vi "TCP - Engine Sender Queue Driver.vi"(6 "timeout(ms)":i32=-1, 7 "Cases":T2, 8 "error in (no error)":errorcluster, 10 "Element In":cluster{"Data":variant, "State":T1}={"Data"=variant, "State"=enum."Boolean Commands"}) -> (0 "error out":errorcluster, 2 "Element Out":cluster{"Data":variant, "State":T1}={"Data"=variant, "State"=enum."Boolean Commands"}, 3 "queue out":refnum<queue>)   [LabVIEW 2017]
uses:
  TCP - Driver Control.ctl
  Controls/RT- Queue States.ctl
panel:
  in  "Enum":T1
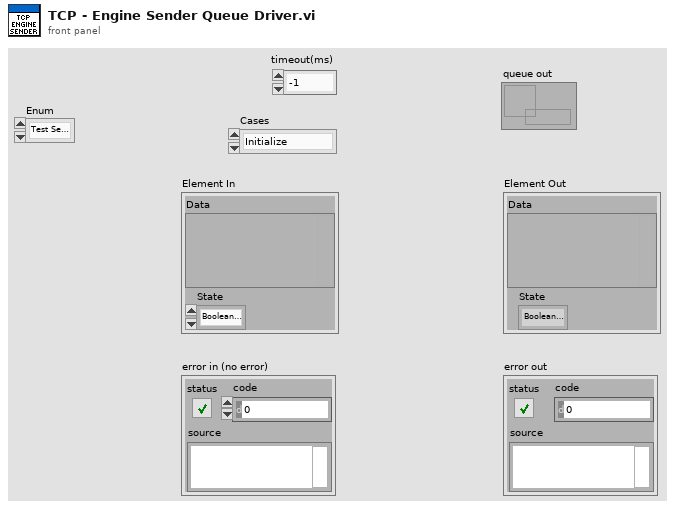
[diagram p1: front panel]
types:
  T1 = typedef "TCP - Driver Control.ctl" = enum16{"Test Settings", "Boolean Commands", "Test Results", "Send Test Details"}
  T2 = typedef "RT- Queue States.ctl" = enum16{"Initialize", "Enqueue", "Enqueue Priority", "Dequeue", "Flush", "Destroy"}
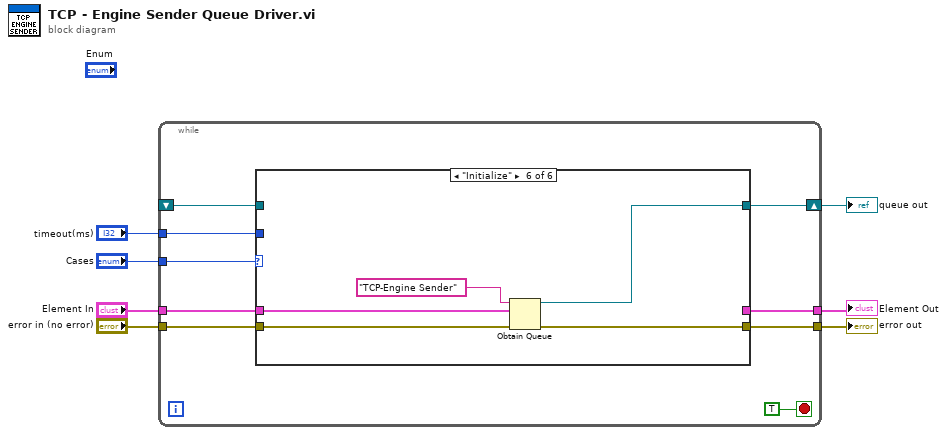
[diagram p0: block diagram]
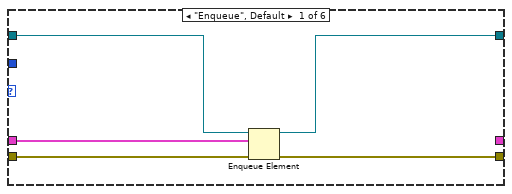
[diagram p2: hidden frame]
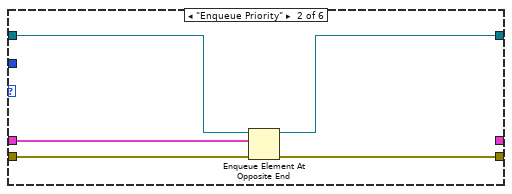
[diagram p3: hidden frame]
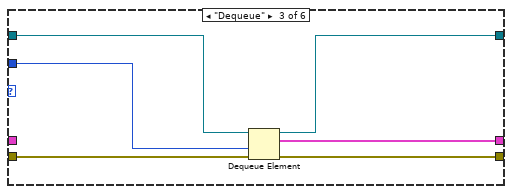
[diagram p4: hidden frame]
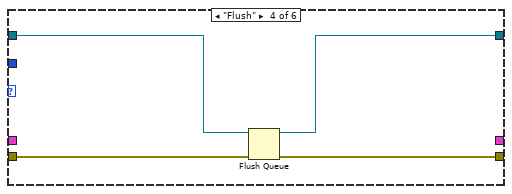
[diagram p5: hidden frame]
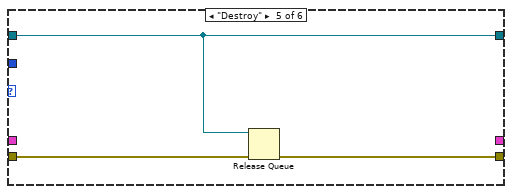
[diagram p6: hidden frame]
diagram:
  n1 = while {
    shift-right: [w15] -> w4
    shift-left: _ -> [w13]
    tunnel: "Cases" -> [w14]
    tunnel: "error in (no error)" -> [w12]
    tunnel: [w11] -> w5
    tunnel: "Element In" -> [w10]
    tunnel: [w9] -> w2
    tunnel: "timeout(ms)" -> [w8]
    stop <- TRUE stop-if-true
    n2 = case shown="\"Initialize\"" w14 {
      tunnel: [w18 w23 w29 w33 w37 w43] -> w15
      tunnel: w13 -> [w19 w24 w30 w34 w37 _]
      tunnel: w12 -> [w21 w26 w32 w36 w39 w42]
      tunnel: [w20 w25 w31 w35 w38 w41] -> w11
      tunnel: w10 -> [w17 w22 _ _ _ w40]
      tunnel: [_ _ w28 _ _ _] -> w9
      tunnel: w8 -> [_ _ w27 _ _ _]
      frame "Enqueue", Default {
        n3 = Enqueue Element(queue=w19, element=w17, error in (no error)=w21) -> (queue out=w18:refnum<queue>, error out=w20:errorcluster)  [unwired: 1 in, 1 out]
      }
      frame "Enqueue Priority" {
        n4 = Enqueue Element At Opposite End(queue=w24, element=w22, error in (no error)=w26) -> (queue out=w23:refnum<queue>, error out=w25:errorcluster)  [unwired: 1 in, 1 out]
      }
      frame "Dequeue" {
        n5 = Dequeue Element(queue=w30, timeout in ms (-1)=w27, error in (no error)=w32) -> (queue out=w29:refnum<queue>, element=w28:cluster{"Data":variant, "State":T1}, error out=w31:errorcluster)  [unwired: 1 out]
      }
      frame "Flush" {
        n6 = Flush Queue(queue=w34, error in (no error)=w36) -> (queue out=w33:refnum<queue>, error out=w35:errorcluster)  [unwired: 1 out]
      }
      frame "Destroy" {
        n7 = Release Queue(queue=w37, error in (no error)=w39) -> (error out=w38:errorcluster)  [unwired: 1 in, 2 out]
      }
      frame "Initialize" {
        n8 = Obtain Queue(name (unnamed)="TCP-Engine Sender", element data type=w40, error in (no error)=w42) -> (queue out=w43:refnum<queue>, error out=w41:errorcluster)  [unwired: 2 in, 1 out]
      }
    }
  }
  "error out" <- w5
  "queue out" <- w4
  "Element Out" <- w2
